vi "find_edge.vi"(10 "q_pulses":i32, 11 "timetags":u32[][](array[numeric])) -> ()   [LabVIEW 2014]
uses:
  <vilib>/Analysis/NI_AALPro.lvlib
  <vilib>/Analysis/NI_AALBase.lvlib
  <vilib>/Analysis/3filter.llb/FIR Filter (DBL).vi
panel:
  out "pulses":u32[](graph)
  out "derivative":dbl[][](graph)
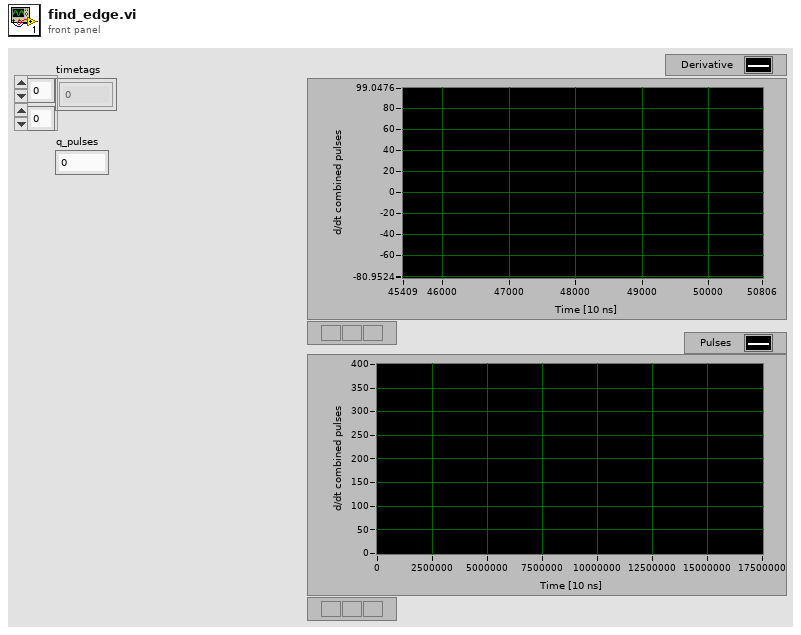
[diagram p1: front panel]
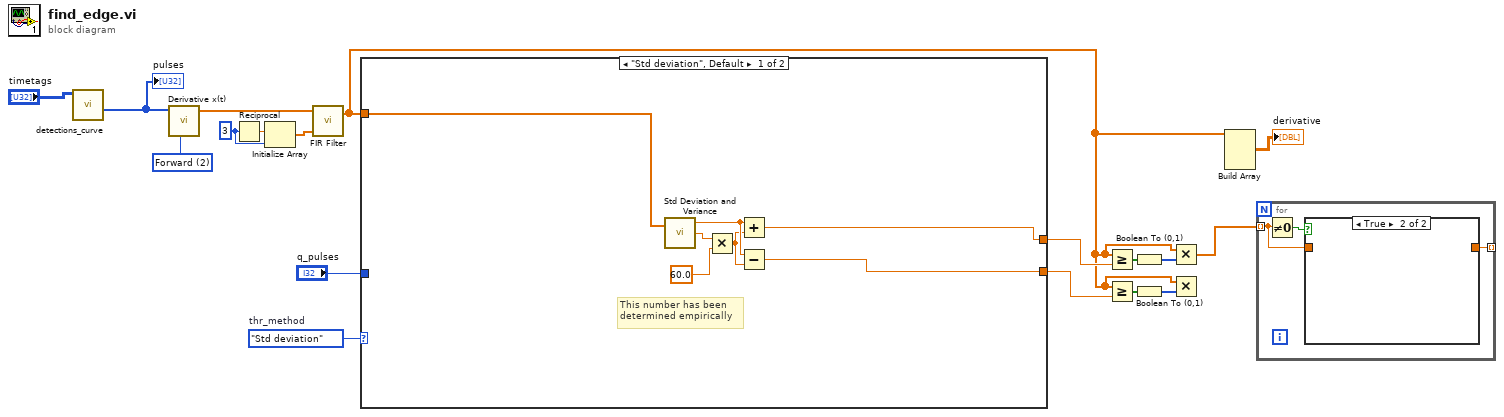
[diagram p0: block diagram]
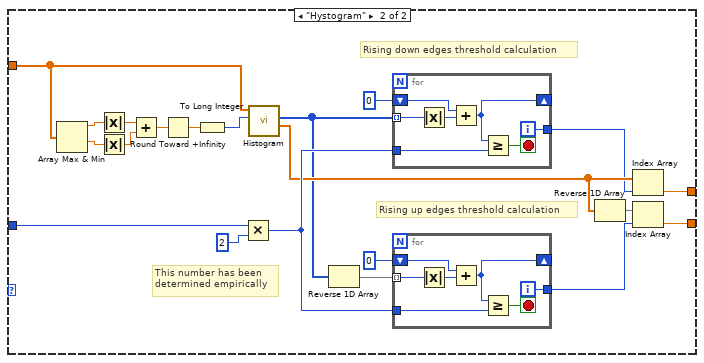
[diagram p3: hidden frame]
diagram:
  w11 = enum16{"Std deviation", "Hystogram"}."Std deviation"  # thr_method
  w15 = 3 ("dimension size")
  w18 = u16 2 items=["2nd Order Central", "4th Order Central", "Forward", "Backward"] ("method")
  n1 = call "detections_curve.vi"("timetags"="timetags") -> ("detections"=w12:u32[])  [unwired: 10 in]
  "pulses" <- w12
  n2 = call <vilib>:"Derivative x(t).vi"("method"=w18, "X"=w12) -> ("dX/dt"=w13:dbl[])  [unwired: 8 in, 1 out]
  n3 = Reciprocal(x=w15) -> (1/x=w17:dbl)
  n4 = Initialize Array(w17, w15) -> (w16:dbl[])
  n5 = call-poly <vilib>:"FIR Filter.vi"("FIR Coefficients"=w16, "X"=w13) -> ("Filtered X"=w2:dbl[])  [unwired: 2 in, 1 out]
  n6 = case shown="\"Std deviation\", Default" w11 {
    tunnel: [w21 w29] -> w9
    tunnel: [w20 w28] -> w3
    tunnel: "q_pulses" -> [_ w27]
    tunnel: w2 -> [w19 w26]
    frame "Std deviation", Default {
      # "This number has been \ndetermined empirically"
      n7 = call <vilib>:"Std Deviation and Variance.vi"("X"=w19) -> ("mean"=w25:dbl, "standard deviation"=w22:dbl)  [unwired: 1 in, 1 out]
      n8 = Multiply(x=w22, y=60.0) -> (x*y=w24:dbl)
      n9 = Add(x=w25, y=w24) -> (x+y=w21:dbl)
      n10 = Subtract(x=w25, y=w24) -> (x-y=w20:dbl)
    }
    frame "Hystogram" {
      # "This number has been \ndetermined empirically"
      # "Rising up edges threshold calculation"
      # "Rising down edges threshold calculation"
      n11 = Array Max & Min(array=w26) -> (max value=w30:dbl, min value=w31:dbl)  [unwired: 2 out]
      n12 = Absolute Value(x=w30) -> (abs(x)=w32:dbl)
      n13 = Absolute Value(x=w31) -> (abs(x)=w33:dbl)
      n14 = Add(x=w32, y=w33) -> (x+y=w34:dbl)
      n15 = Round Toward +Infinity(x=w34) -> (ceil(x): smallest int >= x=w35:dbl)
      n16 = To Long Integer(number=w35) -> (32bit integer=w36:i32)
      n17 = Multiply(x=w27, y=2) -> (x*y=w45:i32)
      n18 = call <vilib>:"Histogram.vi"("intervals"=w36, "X"=w26) -> ("X Values"=w44:dbl[], "Histogram: h(x)"=w40:i32[])  [unwired: 6 in, 2 out]
      n19 = Reverse 1D Array(array=w40) -> (reversed array=w39:i32[])
      n20 = for {
        tunnel: w40 -> [w56] mode=indexing
        shift-right: [w57] -> _
        shift-left: 0 -> [w60]
        tunnel: w45 -> [w59]
        tunnel: [w54] -> w41
        i -> [w54]
        stop <- w58 stop-if-true
        n21 = Absolute Value(x=w56) -> (abs(x)=w55:i32)
        n22 = Add(x=w60, y=w55) -> (x+y=w57:i32)
        n23 = Greater Or Equal?(x=w57, y=w59) -> (x >= y?=w58:bool)
      }
      n24 = for {
        tunnel: w39 -> [w49] mode=indexing
        shift-right: [w50] -> _
        shift-left: 0 -> [w53]
        tunnel: w45 -> [w52]
        tunnel: [w47] -> w42
        i -> [w47]
        stop <- w51 stop-if-true
        n25 = Absolute Value(x=w49) -> (abs(x)=w48:i32)
        n26 = Add(x=w53, y=w48) -> (x+y=w50:i32)
        n27 = Greater Or Equal?(x=w50, y=w52) -> (x >= y?=w51:bool)
      }
      n28 = Reverse 1D Array(array=w44) -> (reversed array=w43:dbl[])
      n29 = Index Array(array=w44, index=w41) -> (element=w29:dbl)
      n30 = Index Array(array=w43, index=w42) -> (element=w28:dbl)
    }
  }
  n31 = Greater Or Equal?(x=w2, y=w9) -> (x >= y?=w7:bool[])
  n32 = Greater Or Equal?(x=w2, y=w3) -> (x >= y?=w5:bool[])
  n33 = Boolean To (0,1)(Boolean=w7) -> (0, 1=w6:i16[])
  n34 = Boolean To (0,1)(Boolean=w5) -> (0, 1=w4:i16[])
  n35 = Multiply(x=w2, y=w6) -> (x*y=w1:dbl[])
  n36 = Multiply(x=w2, y=w4) -> ()  [unwired: 1 out]
  n37 = Build Array(w2) -> (→"derivative":dbl[][])  [unwired: 4 in]
  n38 = for {
    tunnel: w1 -> [w62] mode=indexing
    tunnel: [w61] -> _ mode=indexing
    n39 = Not Equal To 0?(x=w62) -> (x != 0?=w63:bool)
    n40 = case shown="True" w63 {
      tunnel: w62 -> [w64 _]
      tunnel: [w64 _] -> w61
      frame False {
      }
      frame True {
      }
    }
  }
